vi "串口设备参数设置.vi"(8 "布尔文本.文本":string, 9 "section (optional)":string, 10 "监测项描述":string) -> (2 "布尔":bool=TRUE, 3 "输出簇":T2={"监测项描述:输出"="", "连接方式"=enum."串口", "端口"="", "IP address:"="", "Port:"="", "站号"=19200, "传感器型号"="", "波特率"=19200, "data bits"=8, "停止位"=10, "奇偶校验"=0, "声光告警启用"=FALSE} {"data bits" min=5 max=8 step=1; "停止位" items=["1.0"=10, "1.5"=15, "2.0"=20]; "奇偶校验" items=["None", "Odd", "Even", "Mark", "Space"]})   [LabVIEW 2016, in "环境动力监测库.lvlib"]
uses:
  <vilib>/Utility/miscctls.llb/LVPointTypeDef.ctl
  <vilib>/Instr/_visa.llb/VISA Find Search Mode.ctl
  <vilib>/Utility/config.llb/NI_LVConfig.lvlib
panel:
  in  "输出点":T1(ring)
  in  "声光告警启用":bool caption="声光告警"
  in  "参数配置":bool
  in  "连接方式":enum16{"串口", "TCP"}(ring)
  in  "IP address:":string
  in  "Port:":string
  in  "数据比特":u64=8 min=5 max=8 step=1
  in  "波特率":u64=115200
  in  "停止位":u16(ring)=10 items=["1.0"=10, "1.5"=15, "2.0"=20]
  in  "奇偶校验":enum16{"None", "Odd", "Even", "Mark", "Space"}(ring)
  in  "传感器型号":string(combo)
  in  "输入簇":T2={"监测项描述:输出"="", "连接方式"=enum."串口", "端口"="", "IP address:"="", "Port:"="", "站号"=19200, "传感器型号"="", "波特率"=19200, "data bits"=8, "停止位"=10, "奇偶校验"=0, "声光告警启用"=FALSE} {"data bits" min=5 max=8 step=1; "停止位" items=["1.0"=10, "1.5"=15, "2.0"=20]; "奇偶校验" items=["None", "Odd", "Even", "Mark", "Space"]}
  in  "站号":u64=1
  in  "返回":bool
  in  "增加":bool
  in  "端口":u16(ring) items=["COM10", "COM30", "COM3", "COM23", "COM4", "COM24", "COM5", "COM25", "COM6", "COM26", "COM7", "COM27", "COM8", "COM28", "COM9", "COM29", "COM12", "COM11", "COM13", "COM15", "COM16", "COM17", "COM19", "COM20", "COM21", "COM18", "COM31", "COM32", "COM1", "COM2"]
  in  "监测项描述":string
  # "基本设置"
  # "如:红外XX"
  # "传感器选择"
  # "端口选择"
  # "站号配置"
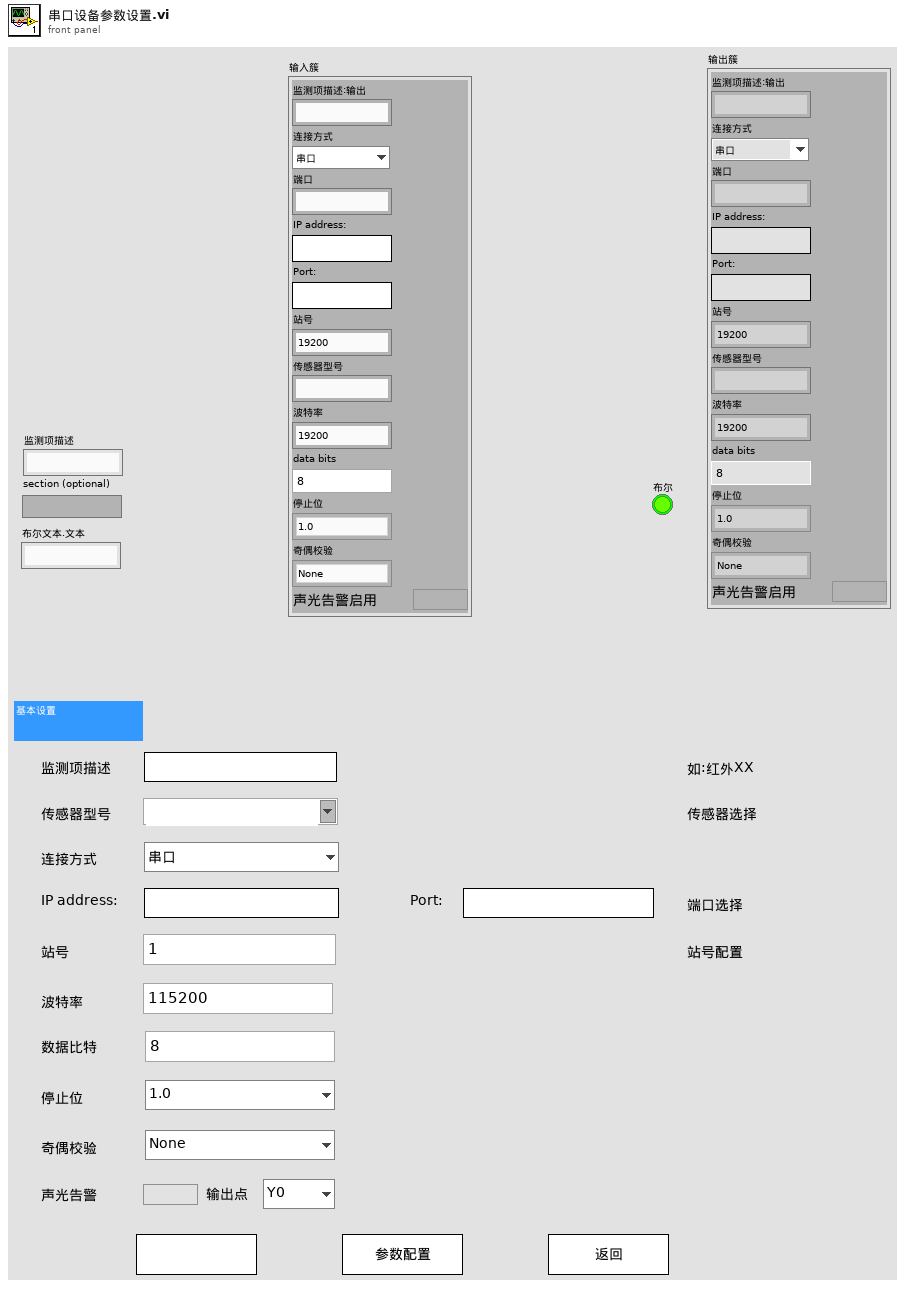
[diagram p1: front panel]
types:
  T1 = enum16{"Y0", "Y1", "Y2", "Y3", "Y4", "Y5", "Y6", "Y7", "Y8", "Y9", "Y10", "Y11", "Y12", "Y13", "Y14", "Y15", "Y16", "Y17", "Y18", "Y19", "Y20", "Y21", "Y22", "Y23", "Y24", "Y25", "Y26", "Y27", "Y28", "Y29", "Y30", "Y31", "Y32", "Y33", "Y34", "Y35", "Y36", "Y37", "Y38", "Y39"}
  T2 = cluster{"监测项描述:输出":string, "连接方式":enum16{"串口", "TCP"}, "端口":string, "IP address:":string, "Port:":string, "站号":u64, "传感器型号":string, "波特率":u64, "data bits":u64, "停止位":u16, "奇偶校验":u16, "声光告警启用":bool}
  T3 = typedef "LVPointTypeDef.ctl" = cluster{"Horizontal":i16, "Vertical":i16}
  T4 = typedef "NI_LVConfig.lvlib/Config Data RefNum.ctl" = refnum<k1>
  T5 = typedef "VISA Find Search Mode.ctl" = u32
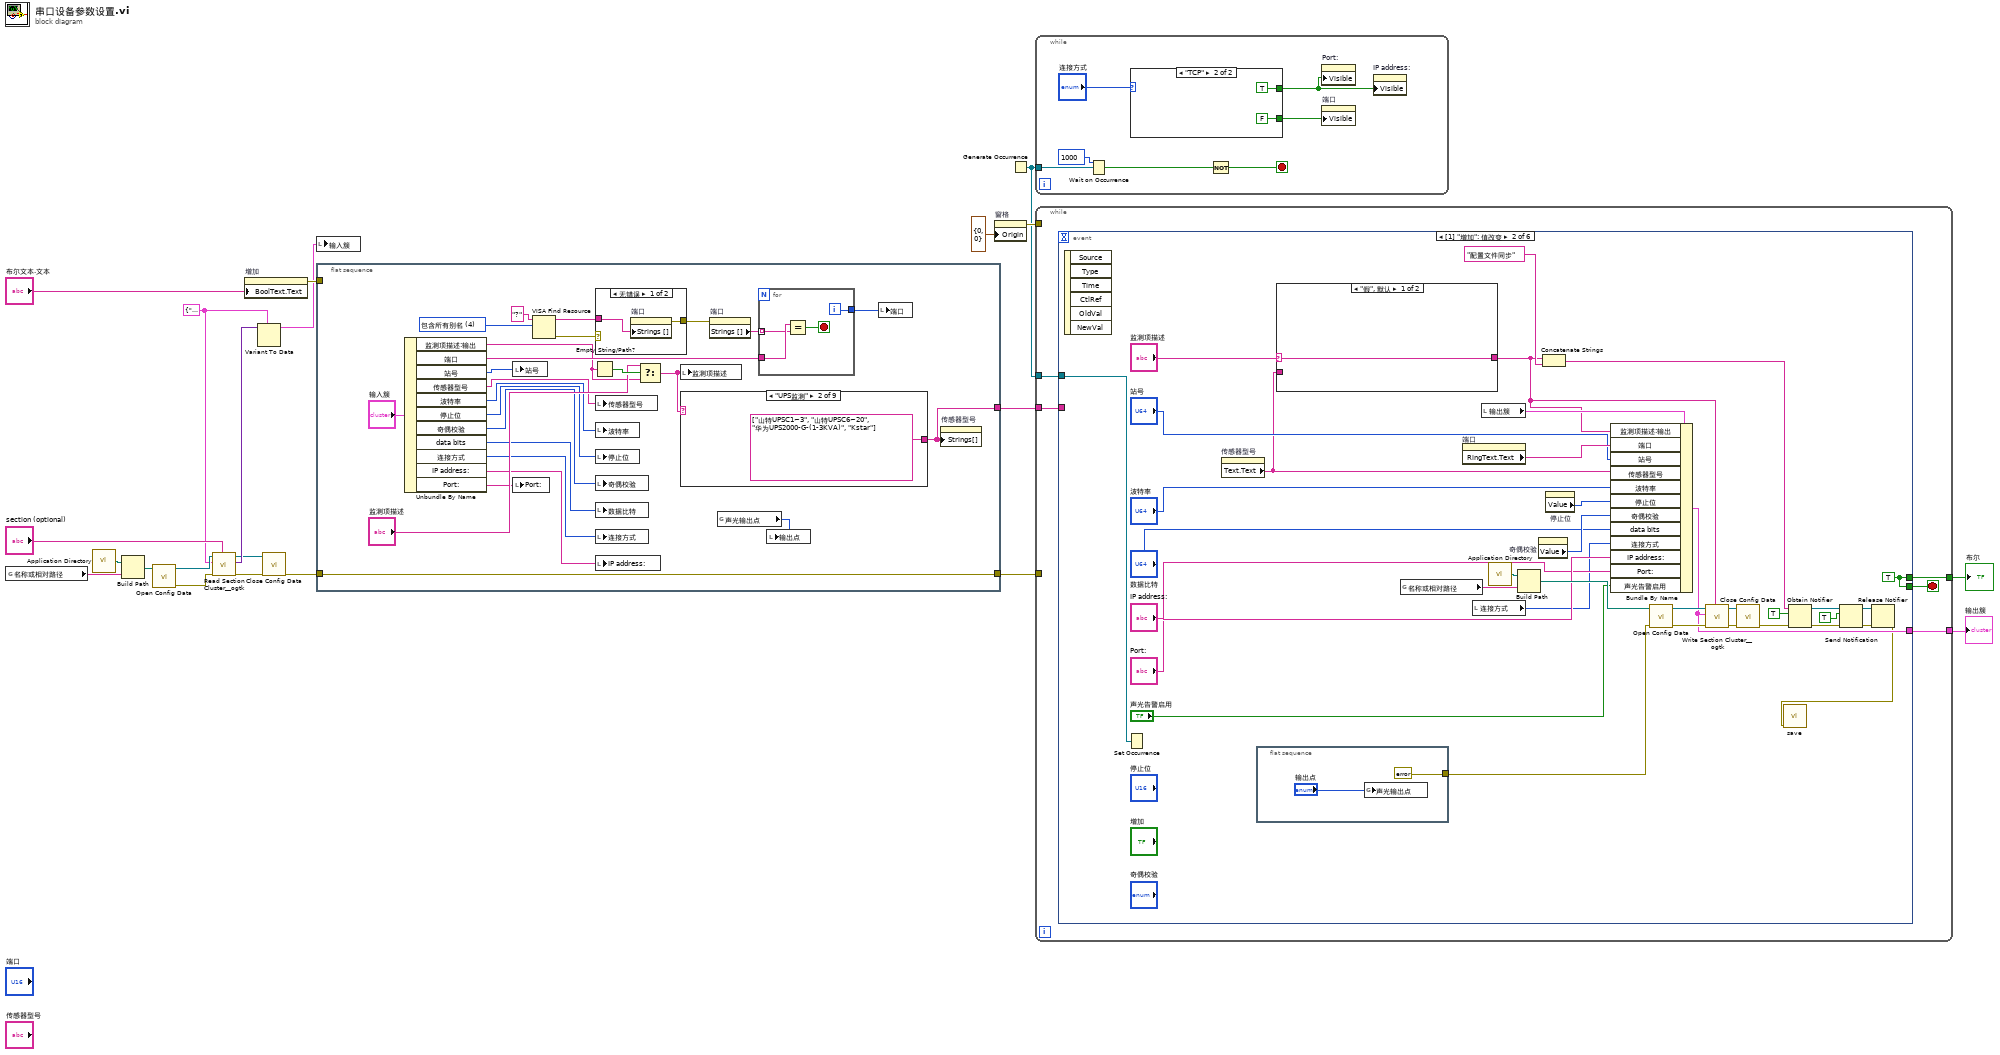
[diagram p0: block diagram]
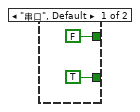
[diagram p2: hidden frame]
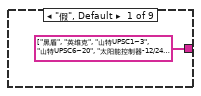
[diagram p4: hidden frame]
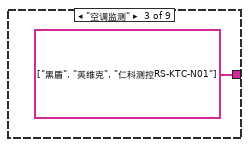
[diagram p5: hidden frame]
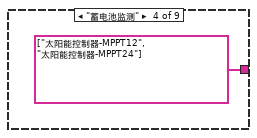
[diagram p6: hidden frame]
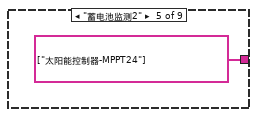
[diagram p7: hidden frame]
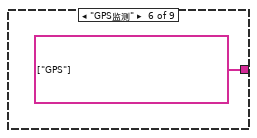
[diagram p8: hidden frame]
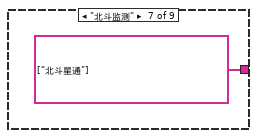
[diagram p9: hidden frame]
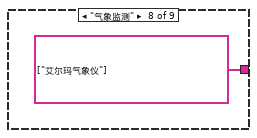
[diagram p10: hidden frame]
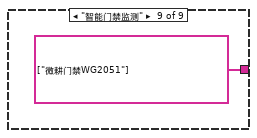
[diagram p11: hidden frame]
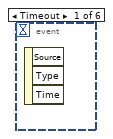
[diagram p12: hidden frame]
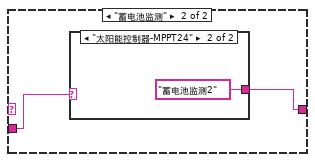
[diagram p13: hidden frame]
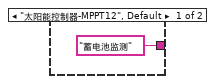
[diagram p14: hidden frame]
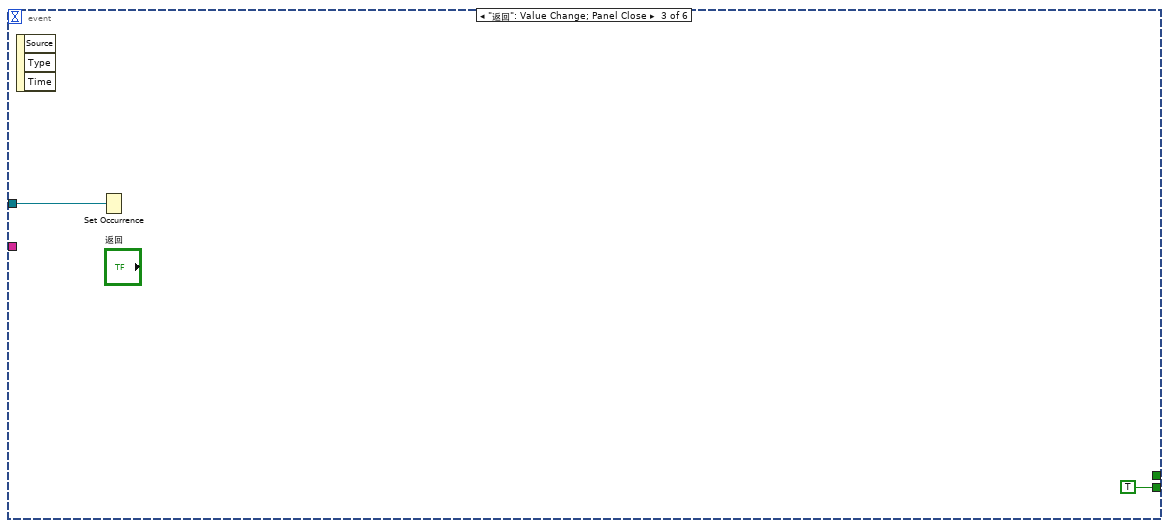
[diagram p15: hidden frame]
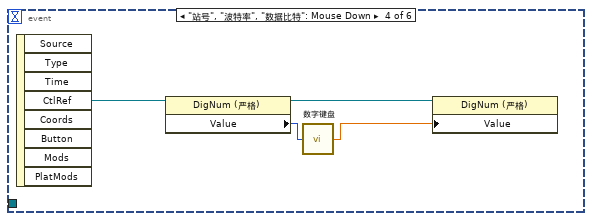
[diagram p16: hidden frame]
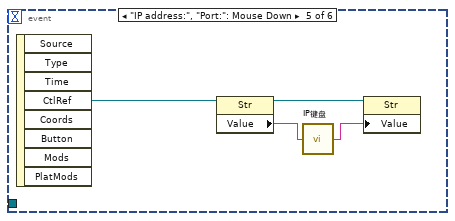
[diagram p17: hidden frame]
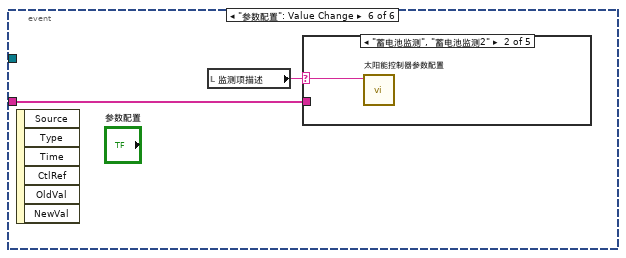
[diagram p18: hidden frame]
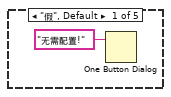
[diagram p19: hidden frame]
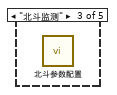
[diagram p20: hidden frame]
diagram:
  w3 = T2 {"监测项描述:输出"="", "连接方式"=enum."串口", "端口"="", "IP address:"="", "Port:"="", "站号"=1, "传感器型号"="", "波特率"=9600, "data bits"=8, "停止位"=10, "奇偶校验"=0, "声光告警启用"=FALSE} ("输入簇")
  n1 = global read "内部交互全局变量.vi" "名称或相对路径"() -> (w1:string)
  n2 = call <vilib>:"Application Directory.vi"() -> ("Application Directory"=w14:path)
  n3 = Build Path(base path=w14, name or relative path=w1) -> (appended path=w15:path)
  n4 = call <vilib>:"Open Config Data.vi"("configuration file path"=w15) -> ("error out"=w16:errorcluster, "refnum"=w17:T4)  [unwired: 8 in, 1 out]
  n5 = call <userlib>:"Read Section Cluster__ogtk.vi"("section (optional)"="section (optional)", "error in (no error)"=w16, "Section Formatted Cluster Type"=w3, "refnum"=w17) -> ("error out"=w10:errorcluster, "Section Formatted Cluster"=w12:variant, "dup refnum"=w11:T4)  [unwired: 3 in, 2 out]
  n6 = property on="增加" class="Bool"("BoolText.Text"="布尔文本.文本") -> (error out=w9:errorcluster)  [unwired: 2 in, 1 out]
  n7 = Variant To Data(type=w3, Variant=w12) -> (data=w2:T2)  [unwired: 1 in, 1 out]
  n8 = call <vilib>:"Close Config Data.vi"("error in (no error)"=w10, "refnum"=w11) -> ("error out"=w8:errorcluster)  [unwired: 8 in, 1 out]
  n9 = local write "输入簇"(w2) -> ()
  n10 = flat-sequence {
    tunnel: w9 -> [_]
    tunnel: w8 -> [w42]
    tunnel: [w42] -> w7
    tunnel: [w28] -> w4
    frame #0 {
      w26 = T5 4 items=["仅允许规范名称"=0, "只允许别名"=2, "包含匹配别名"=3, "包含所有别名"=4] ("Search Mode")
      n11 = Unbundle By Name("输入簇") -> ("监测项描述:输出"=w39:string, "端口"=w45:string, "站号"=w30:u64, "传感器型号"=w38:string, "波特率"=w34:u64, "停止位"=w33:u16, "奇偶校验"=w32:u16, "data bits"=w31:u64, "连接方式"=w37:enum16{"串口", "TCP"}, "IP address:"=w36:string, "Port:"=w35:string)
      n12 = local write "站号"(w30) -> ()
      n13 = local write "Port:"(w35) -> ()
      n14 = VISA Find Resource(10:w26, 11:"?" ("表达式(\"?*\")")) -> (0:w23:errorcluster, 3:w25:string[])  [unwired: 1 in, 1 out]
      n15 = Empty String/Path?(string/path=w39) -> (empty?=w41:bool)
      n16 = case shown="无错误" w23 {
        tunnel: w25 -> [w48 _]
        tunnel: [w47 _] -> w24
        frame No Error {
          n17 = property on="端口" class="Ring (严格)"("Strings []"=w48) -> (error out=w47:errorcluster)  [unwired: 2 in, 1 out]
        }
        frame Error {
        }
      }
      n18 = local write "传感器型号"(w38) -> ()
      n19 = local write "波特率"(w34) -> ()
      n20 = local write "停止位"(w33) -> ()
      n21 = local write "奇偶校验"(w32) -> ()
      n22 = local write "数据比特"(w31) -> ()
      n23 = local write "连接方式"(w37) -> ()
      n24 = local write "IP address:"(w36) -> ()
      n25 = Select(t="监测项描述", s=w41, f=w39) -> (s? t:f=w29:string)
      n26 = local write "监测项描述"(w29) -> ()
      n27 = case shown="\"UPS监测\"" w29 {
        tunnel: [string[] ["黑盾", "英维克", "山特UPSC1~3", "山特UPSC6~20", "太阳能控制器-12/24", "华为UPS2000-G-(1-3KVA)"] ("字符串[]") string[] ["山特UPSC1~3", "山特UPSC6~20", "华为UPS2000-G-(1-3KVA)", "Kstar"] ("字符串[]") string[] ["黑盾", "英维克", "仁科测控RS-KTC-N01"] ("字符串[]") string[] ["太阳能控制器-MPPT12", "太阳能控制器-MPPT24"] ("字符串[]") string[] ["太阳能控制器-MPPT24"] ("字符串[]") string[] ["GPS"] ("字符串[]") string[] ["北斗星通"] ("字符串[]") string[] ["艾尔玛气象仪"] ("字符串[]") string[] ["微耕门禁WG2051"] ("字符串[]")] -> w28
        frame "假", Default {
        }
        frame "UPS监测" {
        }
        frame "空调监测" {
        }
        frame "蓄电池监测" {
        }
        frame "蓄电池监测2" {
        }
        frame "GPS监测" {
        }
        frame "北斗监测" {
        }
        frame "气象监测" {
        }
        frame "智能门禁监测" {
        }
      }
      n28 = property on="端口" class="Ring (严格)"(error in=w24) -> ("Strings []"=w44:string[])  [unwired: 1 in, 2 out]
      n29 = global read "断电保存全局变量.vi" "声光输出点"() -> (w22:T1)
      n30 = for {
        tunnel: w45 -> [w61]
        tunnel: [w59] -> w43
        tunnel: w44 -> [w58] mode=indexing
        i -> [w59]
        stop <- w60 stop-if-true
        n31 = Equal?(x=w61, y=w58) -> (x = y?=w60:bool)
      }
      n32 = local write "输出点"(w22) -> ()
      n33 = local write "端口"(w43) -> ()
      n34 = property on="传感器型号" class="CmbBox"("Strings[]"=w28) -> ()  [unwired: 2 in, 2 out]
    }
  }
  n35 = property on="窗格" class="Pane"("Origin"=T3 {"Horizontal"=0, "Vertical"=0} ("原点")) -> (error out=w21:errorcluster)  [unwired: 2 in, 1 out]
  n36 = Generate Occurrence() -> (w5:refnum<k4>)
  n37 = while {
    tunnel: w5 -> [w68]
    stop <- w65 stop-if-true
    n38 = Wait on Occurrence(2:w68, 3:1000 ("毫秒超时(-1)")) -> (0:w66:bool)  [unwired: 1 in]
    n39 = case shown="\"TCP\"" "连接方式" {
      tunnel: [TRUE FALSE] -> w63
      tunnel: [FALSE TRUE] -> w62
      frame "串口", Default {
      }
      frame "TCP" {
      }
    }
    n40 = Not(x=w66) -> (.not. x?=w65:bool)
    n41 = property on="Port:" class="Str"("Visible"=w62) -> ()  [unwired: 2 in, 2 out]
    n42 = property on="端口" class="Ring (严格)"("Visible"=w63) -> ()  [unwired: 2 in, 2 out]
    n43 = property on="IP address:" class="Str"("Visible"=w62) -> ()  [unwired: 2 in, 2 out]
  }
  n44 = while {
    tunnel: w21 -> [_]
    tunnel: [w77] -> w6
    tunnel: [w75] -> w19
    tunnel: w7 -> [_]
    tunnel: w5 -> [w74]
    tunnel: w4 -> [w73]
    stop <- w76 stop-if-true
    n45 = event shown="[1] \"增加\": 值改变" {
      selector: _ -> [_ _ _ _ _ _]
      dyn-events: _ -> [_ _ _ _ _ _]
      timeout: _ -> [_ _ _ _ _ _]
      tunnel: [_ w106 _ _ _ _] -> w77
      tunnel: [_ w105 TRUE _ _ _] -> w76
      tunnel: [_ w105 _ _ _ _] -> w75
      tunnel: w74 -> [_ w102 w120 _ _ _]
      tunnel: w73 -> [_ _ _ _ _ w130]
      event Timeout {
        n46 = event-data() -> ()  [unwired: 1 in, 3 out]
      }
      event "增加": Value Change {
        w105 = TRUE
        n47 = event-data() -> ()  [unwired: 1 in, 6 out]
        n48 = Set Occurrence(w102) -> ()
        n49 = property on="传感器型号" class="CmbBox"() -> ("Text.Text"=w83:string)  [unwired: 2 in, 2 out]
        n50 = flat-sequence {
          tunnel: [errorcluster {"status"=FALSE, "code"=0, "source"=""} ("error in (no error)")] -> w79
          frame #0 {
            n51 = global write "断电保存全局变量.vi" "声光输出点"("输出点") -> ()
          }
        }
        n52 = case shown="\"假\", 默认" "监测项描述" {
          selector: "监测项描述" -> [w115 _]
          tunnel: w83 -> [_ w117]
          tunnel: [w115 w116] -> w82
          frame "假", Default {
          }
          frame "蓄电池监测" {
            n53 = case shown="\"太阳能控制器-MPPT24\"" w117 {
              tunnel: ["蓄电池监测" ("section (optional)") "蓄电池监测2" ("section (optional)")] -> w116
              frame "太阳能控制器-MPPT12", Default {
              }
              frame "太阳能控制器-MPPT24" {
              }
            }
          }
        }
        n54 = global read "内部交互全局变量.vi" "名称或相对路径"() -> (w80:string)
        n55 = property on="端口" class="Ring (严格)"() -> ("RingText.Text"=w104:string)  [unwired: 2 in, 2 out]
        n56 = local read "连接方式"() -> (w94:enum16{"串口", "TCP"})
        n57 = local read "输出簇"() -> (w101:T2)
        n58 = call <vilib>:"Application Directory.vi"() -> ("Application Directory"=w109:path)
        n59 = Build Path(base path=w109, name or relative path=w80) -> (appended path=w110:path)
        n60 = property on="奇偶校验" class="Enum (严格)"() -> ("Value"=w103:enum16{"None", "Odd", "Even", "Mark", "Space"})  [unwired: 2 in, 2 out]
        n61 = Concatenate Strings(w82, "配置文件同步" ("名称（未命名）")) -> (w85:string)
        n62 = property on="停止位" class="Ring (严格)"() -> ("Value"=w99:u16)  [unwired: 2 in, 2 out]
        n63 = Bundle By Name(cluster=w101, "监测项描述:输出"=w82, "端口"=w104, "站号"="站号", "传感器型号"=w83, "波特率"="波特率", "停止位"=w99, "奇偶校验"=w103, "data bits"="数据比特", "连接方式"=w94, "IP address:"="IP address:", "Port:"="Port:", "声光告警启用"="声光告警启用") -> (w106:T2)
        n64 = call <vilib>:"Open Config Data.vi"("error in (no error)"=w79, "configuration file path"=w110) -> ("error out"=w111:errorcluster, "refnum"=w112:T4)  [unwired: 7 in, 1 out]
        n65 = call <userlib>:"Write Section Cluster__ogtk.vi"("section (optional)"=w82, "error in (no error)"=w111, "Section Formatted Cluster"=w106, "refnum"=w112) -> ("error out"=w107:errorcluster, "dup refnum"=w108:T4)  [unwired: 6 in]
        n66 = call <vilib>:"Close Config Data.vi"("error in (no error)"=w107, "refnum"=w108) -> ("error out"=w90:errorcluster)  [unwired: 8 in, 1 out]
        n67 = Obtain Notifier(name (unnamed)=w85, notification data type=TRUE, error in (no error)=w90) -> (notifier out=w89:refnum<notifier>, error out=w91:errorcluster)  [unwired: 1 in, 1 out]
        n68 = Send Notification(notification=TRUE ("通知"), notifier=w89, error in (no error)=w91) -> (notifier out=w88:refnum<notifier>, error out=w87:errorcluster)
        n69 = Release Notifier(notifier=w88, error in (no error)=w87) -> (error out=w78:errorcluster)  [unwired: 1 in, 2 out]
        n70 = call "save.vi"("error in (no error)"=w78) -> ()  [unwired: 10 in, 1 out]
      }
      event "返回": Value Change; Panel Close {
        n71 = event-data() -> ()  [unwired: 1 in, 3 out]
        n72 = Set Occurrence(w120) -> ()
      }
      event "站号", "波特率", "数据比特": Mouse Down {
        n73 = event-data() -> ("CtlRef"=w125:refnum<vi>)  [unwired: 1 in, 7 out]
        n74 = property class="DigNum (严格)"(reference=w125) -> (reference out=w123:refnum<vi>, "Value"=w124:u64)  [unwired: 1 in, 1 out]
        n75 = call "数字键盘.vi"("OldNumber"=w124) -> ("NewNumber"=w122:sgl)
        n76 = property class="DigNum (严格)"(reference=w123, "Value"=w122) -> ()  [unwired: 1 in, 2 out]
      }
      event "IP address:", "Port:": Mouse Down {
        n77 = event-data() -> ("CtlRef"=w129:refnum<vi>)  [unwired: 1 in, 7 out]
        n78 = property class="Str"(reference=w129) -> (reference out=w128:refnum<vi>, "Value"=w127:string)  [unwired: 1 in, 1 out]
        n79 = call "IP键盘.vi"("OldNumber"=w127) -> ("NewNumber"=w126:string)
        n80 = property class="Str"(reference=w128, "Value"=w126) -> ()  [unwired: 1 in, 2 out]
      }
      event "参数配置": Value Change {
        n81 = event-data() -> ()  [unwired: 1 in, 6 out]
        n82 = local read "监测项描述"() -> (w131:string)
        n83 = case shown="\"蓄电池监测\", \"蓄电池监测2\"" w131 {
          selector: w131 -> [_ w133 _ _ w134]
          tunnel: w130 -> [_ _ _ _ _]
          frame "假", Default {
            n84 = One Button Dialog(message="无需配置!" ("消息")) -> ()  [unwired: 1 in, 1 out]
          }
          frame "蓄电池监测", "蓄电池监测2" {
            n85 = call "太阳能控制器参数配置.vi"("监测项描述"=w133) -> ()  [unwired: 11 in]
          }
          frame "北斗监测" {
            n86 = call "北斗参数配置.vi"() -> ()  [unwired: 12 in]
          }
          frame "GPS监测" {
            n87 = call "GPS参数配置.vi"() -> ()  [unwired: 12 in]
          }
          frame "UPS监测" {
            n88 = call "UPS低电量告警参数配置.vi"("监测项描述"=w134) -> ()  [unwired: 11 in]
          }
        }
      }
    }
  }
  "输出簇" <- w6
  "布尔" <- w19
